vi "74HC74.vi"(6 "R`":bool, 7 "S`":bool, 9 "cp":bool, 10 "D":bool) -> (1 "Q`":bool, 2 "Q":bool)   [LabVIEW 2018]
panel:
  # "上升沿D触发器"
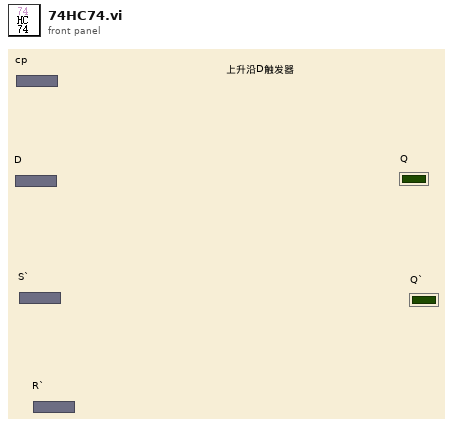
[diagram p1: front panel]
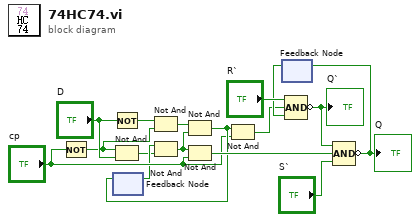
[diagram p0: block diagram]
diagram:
  n1 = Not(x="cp") -> (.not. x?=w1:bool)
  n2 = Not(x="D") -> (.not. x?=w2:bool)
  n3 = Not And(1:"D", 2:w1) -> (0:w5:bool)
  n4 = feedback #1() -> (w6:bool)  [unwired: 1 in]
  n5 = Not And(1:w1, 2:w2) -> (0:w4:bool)
  n6 = Not And(1:w5, 2:w6) -> (0:w8:bool)
  n7 = Not And(1:w8, 2:w4) -> (0:w9:bool)
  n8 = feedback-in #1(w9) -> ()
  n9 = Not And(1:"cp", 2:w8) -> (0:w10:bool)
  n10 = Not And(1:"cp", 2:w9) -> (0:w11:bool)
  n11 = feedback #2() -> (w12:bool)  [unwired: 1 in]
  n12 = Compound Arithmetic op=AND ("复合运算")("R`", w11, w12) -> (invert w14:bool)
  "Q`" <- w14
  n13 = Compound Arithmetic op=AND ("复合运算")(w14, w10, "S`") -> (invert w13:bool)
  "Q" <- w13
  n14 = feedback-in #2(w13) -> ()
